vi "WLAN Common Config.vi"(0 "Instrument Handle In":refnum<k21>, 1 "Selector String":string, 5 "Common Configuration":T1={"Center Frequency (Hz)"=1000000000.0, "Reference Level (dBm)"=0.0, "External Attenuation (dB)"=0.0, "Frequency Reference Source"="OnboardClock", "Digital Edge Source"="PFI0", "Digital Edge"=0, "Trigger Delay (s)"=0.0, "Enable Trigger?"=TRUE, "LO Source"="LO_In", "LO Offset (Hz)"=0.0} {"External Attenuation (dB)" format="%.2f"; "Reference Level (dBm)" format="%.2f"; "Center Frequency (Hz)" format="%.6p"; "Trigger Delay (s)" format="%.3p"; "Digital Edge" items=["Rising Edge", "Falling Edge"]}, 11 "error in (no error)":errorcluster) -> (4 "Instrument Handle Out":refnum<k21>, 15 "error out":errorcluster)   [LabVIEW 2016, in "RFmxWLAN.lvlib"]
uses:
  RFmxWLAN.lvlib
  <resource>/objmgr/RFmxInstr.rc
  <vilib>/RFmx/WLAN/mx/RFmxWLAN.llb/RFmxWLAN Configure Digital Edge Trigger.vi
  Typedefs/WLAN Common Config.ctl
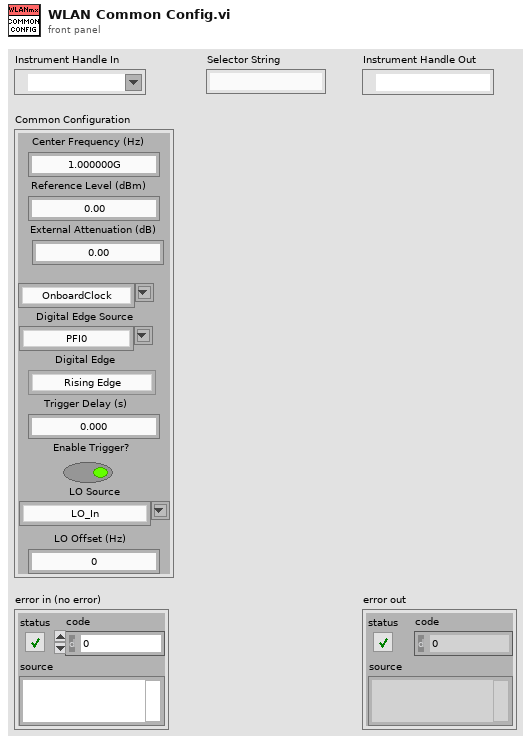
[diagram p1: front panel]
types:
  T1 = typedef "RFmxWLAN.lvlib/WLAN Common Config.ctl" = cluster{"Center Frequency (Hz)":dbl, "Reference Level (dBm)":dbl, "External Attenuation (dB)":dbl, "Frequency Reference Source":string, "Digital Edge Source":string, "Digital Edge":i32, "Trigger Delay (s)":dbl, "Enable Trigger?":bool, "LO Source":string, "LO Offset (Hz)":dbl}
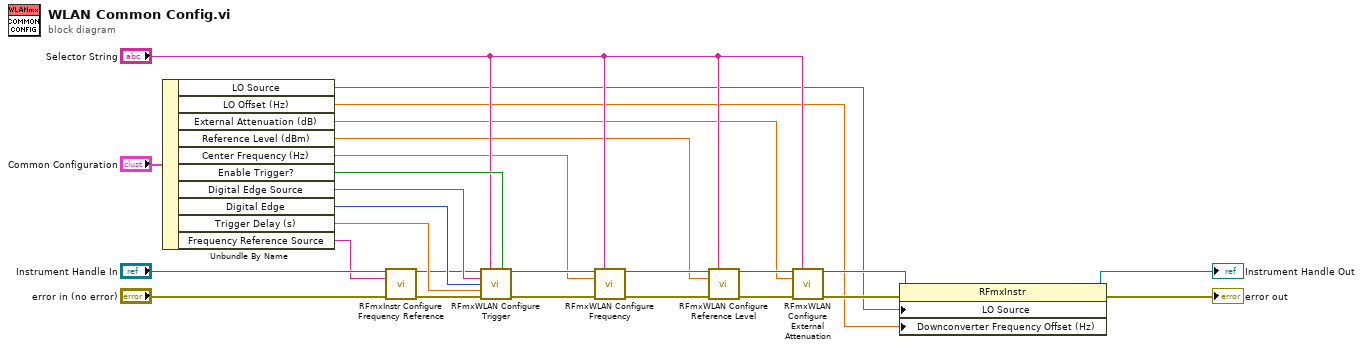
[diagram p0: block diagram]
diagram:
  n1 = Unbundle By Name("Common Configuration") -> ("LO Source"=w2:string, "LO Offset (Hz)"=w1:dbl, "External Attenuation (dB)"=w10:dbl, "Reference Level (dBm)"=w11:dbl, "Center Frequency (Hz)"=w12:dbl, "Enable Trigger?"=w23:bool, "Digital Edge Source"=w22:string, "Digital Edge"=w21:i32, "Trigger Delay (s)"=w20:dbl, "Frequency Reference Source"=w6:string)
  n2 = call <vilib>:"RFmxInstr Configure Frequency Reference.vi"("Instrument Handle In"="Instrument Handle In", "Frequency Reference Source"=w6, "error in (no error)"="error in (no error)") -> ("Instrument Handle Out"=w7:refnum<k21>, "error out"=w9:errorcluster)  [unwired: 11 in]
  n3 = call-poly <vilib>:"RFmxWLAN Configure Trigger.vi"("Instrument Handle In"=w7, "Selector String"="Selector String", "Enable Trigger?"=w23, "Digital Edge Source"=w22, "Digital Edge"=w21, "Trigger Delay (s)"=w20, "error in (no error)"=w9) -> ("Instrument Handle Out"=w17:refnum<k21>, "error out"=w25:errorcluster)  [unwired: 7 in]
  n4 = call <vilib>:"RFmxWLAN Configure Frequency.vi"("Instrument Handle In"=w17, "Selector String"="Selector String", "Center Frequency (Hz)"=w12, "error in (no error)"=w25) -> ("Instrument Handle Out"=w16:refnum<k21>, "error out"=w18:errorcluster)  [unwired: 10 in]
  n5 = call <vilib>:"RFmxWLAN Configure Reference Level.vi"("Instrument Handle In"=w16, "Selector String"="Selector String", "Reference Level"=w11, "error in (no error)"=w18) -> ("Instrument Handle Out"=w14:refnum<k21>, "error out"=w19:errorcluster)  [unwired: 10 in]
  n6 = call <vilib>:"RFmxWLAN Configure External Attenuation.vi"("Instrument Handle In"=w14, "Selector String"="Selector String", "External Attenuation (dB)"=w10, "error in (no error)"=w19) -> ("Instrument Handle Out"=w4:refnum<k21>, "error out"=w15:errorcluster)  [unwired: 10 in]
  n7 = property class="RFmxInstr"(reference=w4, error in=w15, "LO Source"=w2, "Downconverter Frequency Offset (Hz)"=w1) -> (reference out=→"Instrument Handle Out":refnum<k21>, error out=→"error out":errorcluster)
